vi "initalise.vi"(8 "error in (no error)":errorcluster, 9 "Hardware Connected?":bool, 10 "Camera":enum16{"AndorIKon", "ICCamera"}(ring)=enum."ICCamera") -> (0 "error out":errorcluster, 3 "CameraManager out":refnum<class "CameraManager.lvclass">)   [LabVIEW 2011, in "iManagement.lvlib" / "CameraManager.lvclass"]
uses:
  CameraManager.lvclass
  CameraManager.lvclass/CameraManager.ctl
  Hal/Channels/Camera/CameraTempController.lvclass
  Hal/Channels/Camera/CameraSettingsManager/CameraSettingsManager.lvclass
  Tools/SettingsManager/SettingsManager.lvclass
  Hal/Channels/Camera/ICCamera/ICSettingsViewer/ICSettingsViewer.lvclass
  Tools/SettingsViewer/settingsViewer.lvclass
  Hal/Channels/Camera/CameraSettingsEventsManager/cameraSettingsEventManager.lvclass
  Tools/SettingsEventManager/SettingsEventsManager.lvclass
  Hal/Channels/Camera/CameraEventsManager/CameraEventsManger.lvclass
  Hal/Channels/Camera/CameraAcquisitor.lvclass
  Hal/Channels/Camera/CameraController.lvclass
  Hal/Channels/Camera/ICCamera/ICCameraAcquisitor/ICCameraAcquisitor.lvclass
  Hal/Channels/Camera/ICCamera/ICCameraController/ICCameraController.lvclass
  Hal/Channels/Camera/AndorIKonTempController.lvclass
  Hal/Channels/Camera/CameraSettingsViewer/andorSettingsViewer.lvclass
  Hal/Channels/Camera/AndorIKonAcquisitor.lvclass
  Hal/Channels/Camera/AndorController.lvclass
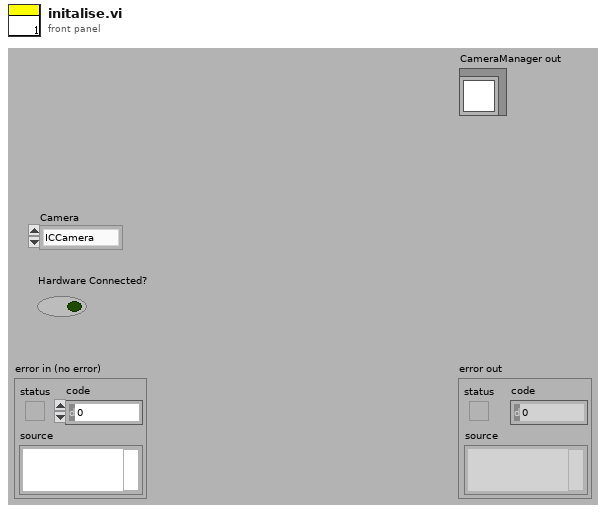
[diagram p1: front panel]
types:
  T1 = cluster{"newSetPointEvent":refnum<user-event>, "stopCoolingEvent":refnum<user-event>}
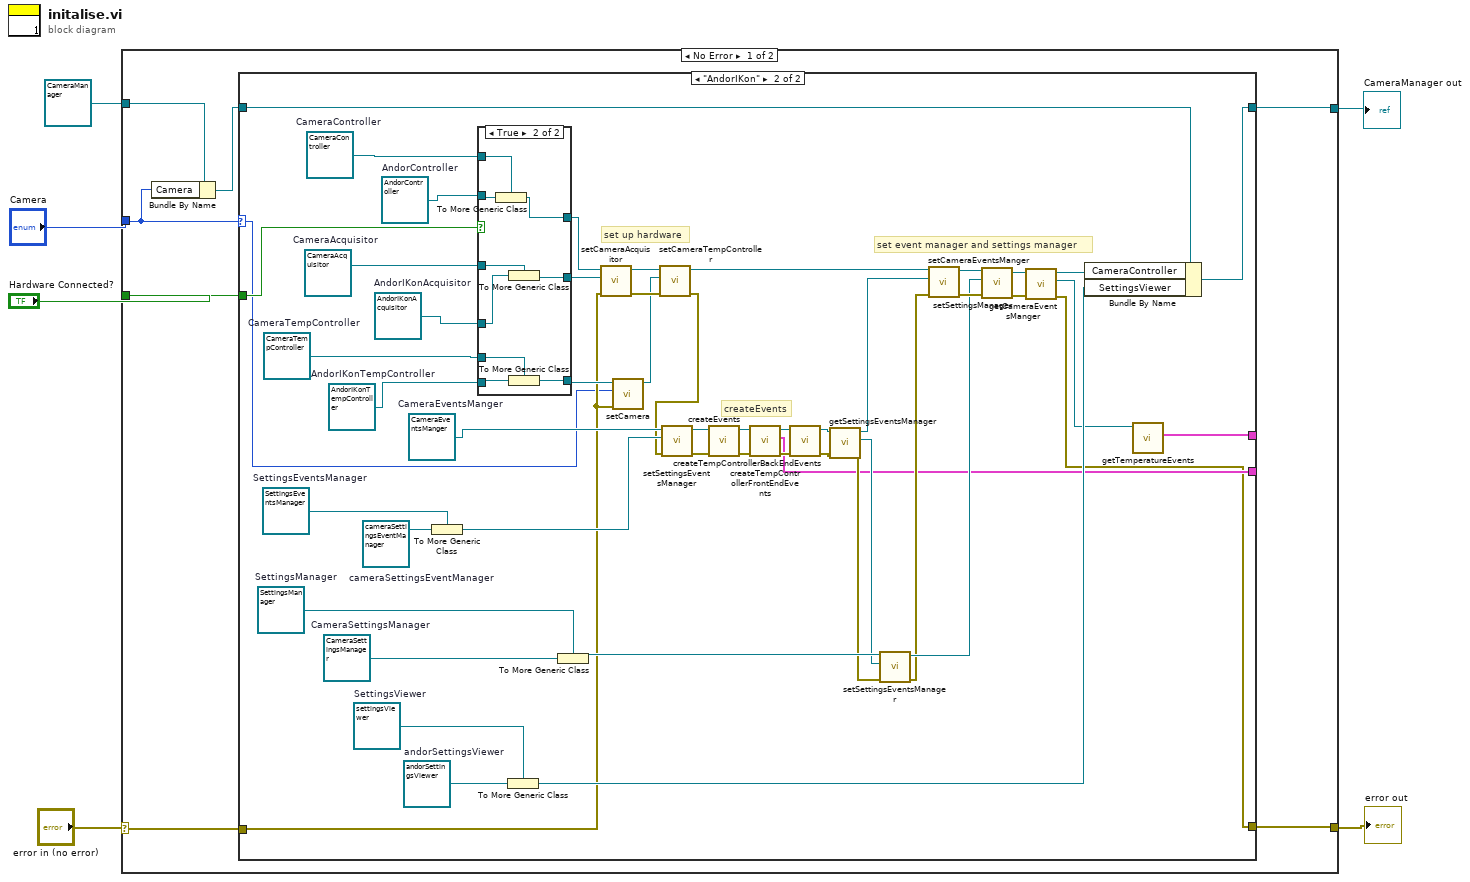
[diagram p0: block diagram]
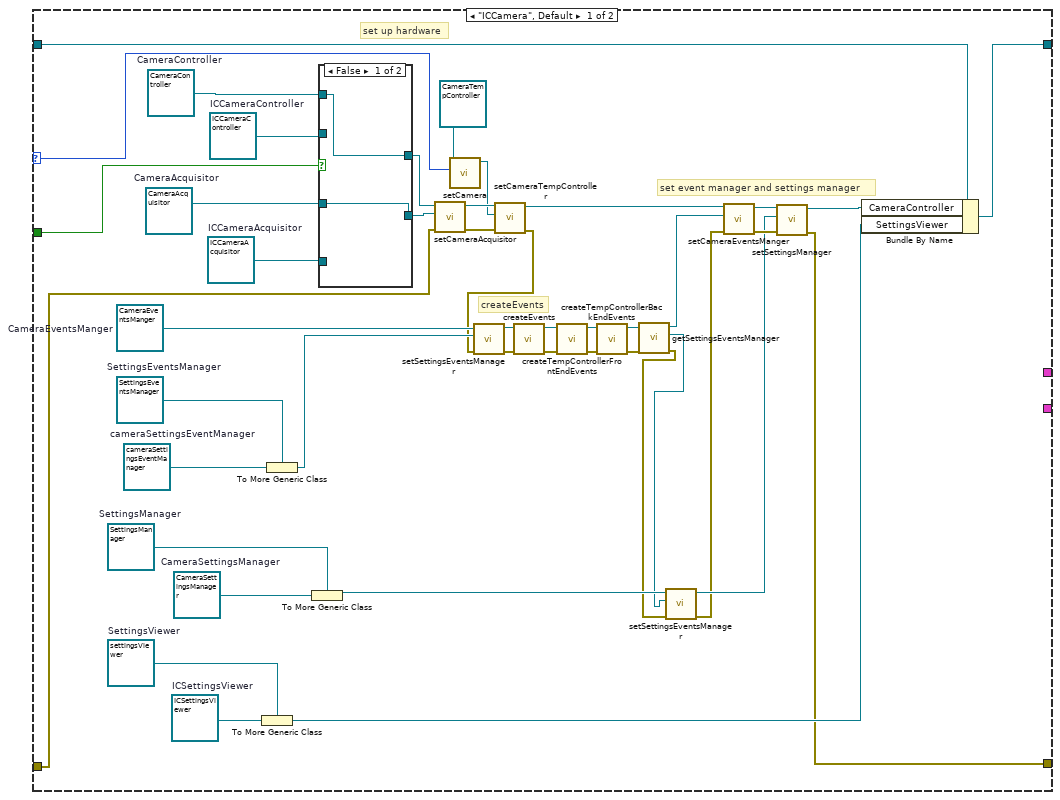
[diagram p2: hidden frame]
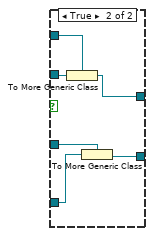
[diagram p3: hidden frame]
diagram:
  n1 = case shown="No Error" "error in (no error)" {
    selector: "error in (no error)" -> [w13 w129]
    tunnel: [w12 w129] -> w5
    tunnel: [w11 _] -> w4
    tunnel: "Camera" -> [w9 _]
    tunnel: "Hardware Connected?" -> [w10 _]
    tunnel: refnum<class "CameraManager.lvclass"> refnum ("iManagement.lvlib:CameraManager.lvclass") -> [w8 _]
    frame No Error {
      n2 = Bundle By Name(cluster=w8, "Camera"=w9) -> (w7:refnum<class "CameraManager.lvclass">)
      n3 = case shown="\"AndorIKon\"" w9 {
        selector: w9 -> [w20 w79]
        tunnel: w13 -> [w41 w80]
        tunnel: [w27 w68] -> w12
        tunnel: w7 -> [w31 w94]
        tunnel: [w28 w92] -> w11
        tunnel: w10 -> [w51 w112]
        tunnel: [_ w72] -> _
        tunnel: [_ w66] -> _
        frame "ICCamera", Default {
          w44 = refnum<class "CameraSettingsManager.lvclass"> refnum  # CameraSettingsManager
          w43 = refnum<class "SettingsManager.lvclass"> refnum  # SettingsManager
          w42 = refnum<class "ICSettingsViewer.lvclass"> refnum  # ICSettingsViewer
          w40 = refnum<class "settingsViewer.lvclass"> refnum  # SettingsViewer
          w50 = refnum<class "cameraSettingsEventManager.lvclass"> refnum  # cameraSettingsEventManager
          w45 = refnum<class "SettingsEventsManager.lvclass"> refnum  # SettingsEventsManager
          w46 = refnum<class "CameraEventsManger.lvclass"> refnum  # CameraEventsManger
          w55 = refnum<class "CameraAcquisitor.lvclass"> refnum  # CameraAcquisitor
          w57 = refnum<class "CameraController.lvclass"> refnum  # CameraController
          w52 = refnum<class "ICCameraAcquisitor.lvclass"> refnum  # ICCameraAcquisitor
          w53 = refnum<class "ICCameraController.lvclass"> refnum  # ICCameraController
          # "set event manager and settings manager"
          # "createEvents"
          # "set up hardware"
          n4 = To More Generic Class(target class=w40, reference=w42) -> (generic class reference=w29:refnum<class "settingsViewer.lvclass">)
          n5 = To More Generic Class(target class=w45, reference=w50) -> (generic class reference=w49:refnum<class "SettingsEventsManager.lvclass">)
          n6 = To More Generic Class(target class=w43, reference=w44) -> (generic class reference=w39:refnum<class "SettingsManager.lvclass">)
          n7 = case shown="False" w51 {
            tunnel: w53 -> [_ w65]
            tunnel: w57 -> [w59 w64]
            tunnel: [w59 w63] -> w56
            tunnel: w55 -> [w58 w62]
            tunnel: [w58 w60] -> w54
            tunnel: w52 -> [_ w61]
            frame False {
            }
            frame True {
              n8 = To More Generic Class(target class=w64, reference=w65) -> (generic class reference=w63:refnum<class "CameraController.lvclass">)
              n9 = To More Generic Class(target class=w62, reference=w61) -> (generic class reference=w60:refnum<class "CameraAcquisitor.lvclass">)
            }
          }
          n10 = call-dynamic "setCameraAcquisitor.vi"("error in (no error)"=w41, "Hardware:Channels.lvlib:CameraAcquisitor.lvclass"=w54, "CameraController.lvclass in"=w56) -> ("error out"=w22:errorcluster, "CameraController.lvclass out"=w25:refnum<class "CameraController.lvclass">)  [unwired: 7 in]
          n11 = call-dynamic "setCamera.vi"("Camera"=w20, "CameraTempController.lvclass in"=refnum<class "CameraTempController.lvclass"> refnum) -> ("CameraTempController.lvclass out"=w24:refnum<class "CameraTempController.lvclass">)  [unwired: 8 in, 1 out]
          n12 = call-dynamic "setCameraTempController.vi"("error in (no error)"=w22, "Hardware:Channels.lvlib:CameraTempController.lvclass"=w24, "CameraController.lvclass in"=w25) -> ("error out"=w21:errorcluster, "CameraController.lvclass out"=w23:refnum<class "CameraController.lvclass">)  [unwired: 7 in]
          n13 = call-dynamic "setSettingsEventsManager.vi"("error in (no error)"=w21, "Tools.lvlib:Settings.lvlib:SettingsEventsManager.lvclass"=w49, "CameraEventsManger.lvclass in"=w46) -> ("error out"=w47:errorcluster, "CameraEventsManger.lvclass out"=w48:refnum<class "CameraEventsManger.lvclass">)  [unwired: 7 in]
          n14 = call-dynamic "createEvents.vi"("error in (no error)"=w47, "CameraEventsManger in"=w48) -> ("error out"=w18:errorcluster, "CameraEventsManger out"=w17:refnum<class "CameraEventsManger.lvclass">)  [unwired: 8 in]
          n15 = call-dynamic "createTempControllerFrontEndEvents.vi"("error in (no error)"=w18, "CameraEventsManger.lvclass in"=w17) -> ("error out"=w19:errorcluster, "CameraEventsManger.lvclass out"=w16:refnum<class "CameraEventsManger.lvclass">)  [unwired: 7 in, 1 out]
          n16 = call-dynamic "createTempControllerBackEndEvents.vi"("error in (no error)"=w19, "CameraEventsManger.lvclass in"=w16) -> ("error out"=w15:errorcluster, "CameraEventsManger.lvclass out"=w14:refnum<class "CameraEventsManger.lvclass">)  [unwired: 7 in, 1 out]
          n17 = call-dynamic "getSettingsEventsManager.vi"("error in (no error)"=w15, "CameraEventsManger.lvclass in"=w14) -> ("error out"=w37:errorcluster, "SettingsEventsManager"=w38:refnum<class "SettingsEventsManager.lvclass">, "CameraEventsManger.lvclass out"=w33:refnum<class "CameraEventsManger.lvclass">)  [unwired: 7 in]
          n18 = call-dynamic "setSettingsEventsManager.vi"("error in (no error)"=w37, "Tools.lvlib:Settings.lvlib:SettingsEventsManager.lvclass"=w38, "SettingsManager.lvclass in"=w39) -> ("error out"=w32:errorcluster, "SettingsManager.lvclass out"=w34:refnum<class "SettingsManager.lvclass">)  [unwired: 7 in]
          n19 = call-dynamic "setCameraEventsManger.vi"("error in (no error)"=w32, "Hardware:Channels.lvlib:CameraEventsManger.lvclass"=w33, "CameraController.lvclass in"=w23) -> ("error out"=w35:errorcluster, "CameraController.lvclass out"=w36:refnum<class "CameraController.lvclass">)  [unwired: 7 in]
          n20 = call-dynamic "setSettingsManager.vi"("error in (no error)"=w35, "Tools.lvlib:Settings.lvlib:SettingsManager.lvclass"=w34, "CameraController.lvclass in"=w36) -> ("error out"=w27:errorcluster, "CameraController.lvclass out"=w30:refnum<class "CameraController.lvclass">)  [unwired: 7 in]
          n21 = Bundle By Name(cluster=w31, "CameraController"=w30, "SettingsViewer"=w29) -> (w28:refnum<class "CameraManager.lvclass">)
        }
        frame "AndorIKon" {
          w87 = refnum<class "AndorIKonTempController.lvclass"> refnum  # AndorIKonTempController
          w88 = refnum<class "CameraTempController.lvclass"> refnum  # CameraTempController
          w89 = refnum<class "andorSettingsViewer.lvclass"> refnum  # andorSettingsViewer
          w91 = refnum<class "AndorIKonAcquisitor.lvclass"> refnum  # AndorIKonAcquisitor
          w90 = refnum<class "AndorController.lvclass"> refnum  # AndorController
          w105 = refnum<class "CameraSettingsManager.lvclass"> refnum  # CameraSettingsManager
          w104 = refnum<class "SettingsManager.lvclass"> refnum  # SettingsManager
          w103 = refnum<class "settingsViewer.lvclass"> refnum  # SettingsViewer
          w111 = refnum<class "cameraSettingsEventManager.lvclass"> refnum  # cameraSettingsEventManager
          w106 = refnum<class "SettingsEventsManager.lvclass"> refnum  # SettingsEventsManager
          w107 = refnum<class "CameraEventsManger.lvclass"> refnum  # CameraEventsManger
          w114 = refnum<class "CameraAcquisitor.lvclass"> refnum  # CameraAcquisitor
          w116 = refnum<class "CameraController.lvclass"> refnum  # CameraController
          # "set event manager and settings manager"
          # "createEvents"
          # "set up hardware"
          n22 = To More Generic Class(target class=w106, reference=w111) -> (generic class reference=w110:refnum<class "SettingsEventsManager.lvclass">)
          n23 = case shown="True" w112 {
            tunnel: w90 -> [_ w128]
            tunnel: w116 -> [w119 w127]
            tunnel: [w119 w126] -> w115
            tunnel: w114 -> [w118 w125]
            tunnel: [w118 w123] -> w113
            tunnel: w91 -> [_ w124]
            tunnel: w88 -> [w117 w122]
            tunnel: w87 -> [_ w121]
            tunnel: [w117 w120] -> w82
            frame False {
            }
            frame True {
              n24 = To More Generic Class(target class=w127, reference=w128) -> (generic class reference=w126:refnum<class "CameraController.lvclass">)
              n25 = To More Generic Class(target class=w125, reference=w124) -> (generic class reference=w123:refnum<class "CameraAcquisitor.lvclass">)
              n26 = To More Generic Class(target class=w122, reference=w121) -> (generic class reference=w120:refnum<class "CameraTempController.lvclass">)
            }
          }
          n27 = To More Generic Class(target class=w103, reference=w89) -> (generic class reference=w93:refnum<class "settingsViewer.lvclass">)
          n28 = To More Generic Class(target class=w104, reference=w105) -> (generic class reference=w102:refnum<class "SettingsManager.lvclass">)
          n29 = call-dynamic "setCameraAcquisitor.vi"("error in (no error)"=w80, "Hardware:Channels.lvlib:CameraAcquisitor.lvclass"=w113, "CameraController.lvclass in"=w115) -> ("error out"=w85:errorcluster, "CameraController.lvclass out"=w86:refnum<class "CameraController.lvclass">)  [unwired: 7 in]
          n30 = call-dynamic "setCamera.vi"("error in (no error)"=w80, "Camera"=w79, "CameraTempController.lvclass in"=w82) -> ("CameraTempController.lvclass out"=w81:refnum<class "CameraTempController.lvclass">)  [unwired: 7 in, 1 out]
          n31 = call-dynamic "setCameraTempController.vi"("error in (no error)"=w85, "Hardware:Channels.lvlib:CameraTempController.lvclass"=w81, "CameraController.lvclass in"=w86) -> ("error out"=w84:errorcluster, "CameraController.lvclass out"=w83:refnum<class "CameraController.lvclass">)  [unwired: 7 in]
          n32 = call-dynamic "setSettingsEventsManager.vi"("error in (no error)"=w84, "Tools.lvlib:Settings.lvlib:SettingsEventsManager.lvclass"=w110, "CameraEventsManger.lvclass in"=w107) -> ("error out"=w108:errorcluster, "CameraEventsManger.lvclass out"=w109:refnum<class "CameraEventsManger.lvclass">)  [unwired: 7 in]
          n33 = call-dynamic "createEvents.vi"("error in (no error)"=w108, "CameraEventsManger in"=w109) -> ("error out"=w75:errorcluster, "CameraEventsManger out"=w76:refnum<class "CameraEventsManger.lvclass">)  [unwired: 8 in]
          n34 = call-dynamic "createTempControllerFrontEndEvents.vi"("error in (no error)"=w75, "CameraEventsManger.lvclass in"=w76) -> ("error out"=w78:errorcluster, "tempControllerFrontEndEvents"=w72:T1, "CameraEventsManger.lvclass out"=w77:refnum<class "CameraEventsManger.lvclass">)  [unwired: 7 in]
          n35 = call-dynamic "createTempControllerBackEndEvents.vi"("error in (no error)"=w78, "CameraEventsManger.lvclass in"=w77) -> ("error out"=w73:errorcluster, "CameraEventsManger.lvclass out"=w74:refnum<class "CameraEventsManger.lvclass">)  [unwired: 7 in, 1 out]
          n36 = call-dynamic "getSettingsEventsManager.vi"("error in (no error)"=w73, "CameraEventsManger.lvclass in"=w74) -> ("error out"=w100:errorcluster, "SettingsEventsManager"=w101:refnum<class "SettingsEventsManager.lvclass">, "CameraEventsManger.lvclass out"=w96:refnum<class "CameraEventsManger.lvclass">)  [unwired: 7 in]
          n37 = call-dynamic "setSettingsEventsManager.vi"("error in (no error)"=w100, "Tools.lvlib:Settings.lvlib:SettingsEventsManager.lvclass"=w101, "SettingsManager.lvclass in"=w102) -> ("error out"=w95:errorcluster, "SettingsManager.lvclass out"=w97:refnum<class "SettingsManager.lvclass">)  [unwired: 7 in]
          n38 = call-dynamic "setCameraEventsManger.vi"("error in (no error)"=w95, "Hardware:Channels.lvlib:CameraEventsManger.lvclass"=w96, "CameraController.lvclass in"=w83) -> ("error out"=w98:errorcluster, "CameraController.lvclass out"=w99:refnum<class "CameraController.lvclass">)  [unwired: 7 in]
          n39 = call-dynamic "setSettingsManager.vi"("error in (no error)"=w98, "Tools.lvlib:Settings.lvlib:SettingsManager.lvclass"=w97, "CameraController.lvclass in"=w99) -> ("error out"=w69:errorcluster, "CameraController.lvclass out"=w71:refnum<class "CameraController.lvclass">)  [unwired: 7 in]
          n40 = call-dynamic "getCameraEventsManger.vi"("error in (no error)"=w69, "CameraController.lvclass in"=w71) -> ("error out"=w68:errorcluster, "Hardware:Channels.lvlib:CameraEventsManger.lvclass"=w67:refnum<class "CameraEventsManger.lvclass">, "CameraController.lvclass out"=w70:refnum<class "CameraController.lvclass">)  [unwired: 7 in]
          n41 = Bundle By Name(cluster=w94, "CameraController"=w70, "SettingsViewer"=w93) -> (w92:refnum<class "CameraManager.lvclass">)
          n42 = call-dynamic "getTemperatureEvents.vi"("CameraEventsManger.lvclass in"=w67) -> ("temperatureEvents"=w66:T1)  [unwired: 8 in, 2 out]
        }
      }
    }
    frame Error {
    }
  }
  "error out" <- w5
  "CameraManager out" <- w4
